vi "Read Measurement Type.vi"(8 "error in":errorcluster, 11 "PWM input channel in":refnum<class "PWM Input Channel.lvclass">) -> (0 "error out":errorcluster, 2 "measurement type":T1, 3 "PWM input channel out":refnum<class "PWM Input Channel.lvclass">)   [LabVIEW 2017, in "Scan Engine Scripting.lvlib" / "PWM Input Channel.lvclass"]
uses:
  PWM Input Channel.lvclass
  Measurement Type.ctl
  PWM Input Channel.lvclass/PWM Input Channel.ctl
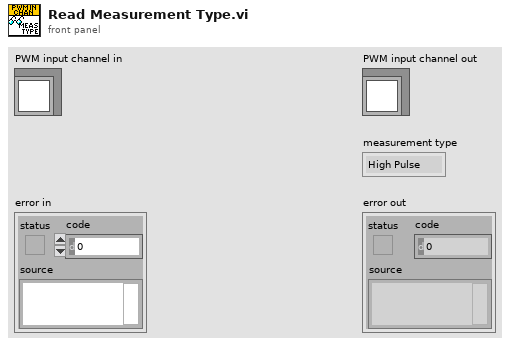
[diagram p1: front panel]
types:
  T1 = typedef "Scan Engine Scripting.lvlib/PWM Input Channel.lvclass/Measurement Type.ctl" = enum16{"High Pulse", "Low Pulse", "Most Recent"}
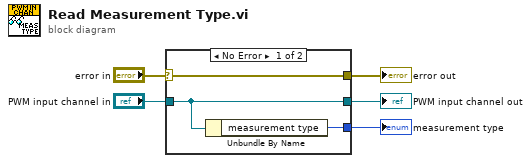
[diagram p0: block diagram]
diagram:
  n1 = case shown="No Error" "error in" {
    selector: "error in" -> [w8 w9]
    tunnel: [w8 w9] -> w4
    tunnel: [w7 w10] -> w2
    tunnel: "PWM input channel in" -> [w7 w10]
    tunnel: [w6 _] -> w1
    frame No Error {
      n2 = Unbundle By Name(w7) -> ("measurement type"=w6:T1)
    }
    frame Error {
    }
  }
  "error out" <- w4
  "PWM input channel out" <- w2
  "measurement type" <- w1
